vi "shift_register.vi"() -> ()   [LabVIEW 2020]
panel:
  out "Cluster":cluster{"array bool":bool[], "array num":dbl[]}
  out "Array":bool[](array[boolean])
  out "Boolean 2":bool
  out "concatenated string":string
  out "Numeric 2":u16
  in  "stop":bool
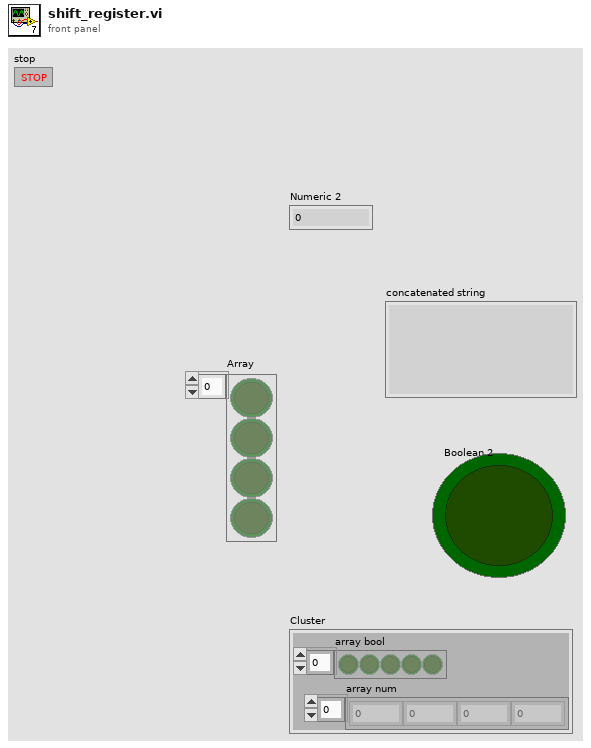
[diagram p1: front panel]
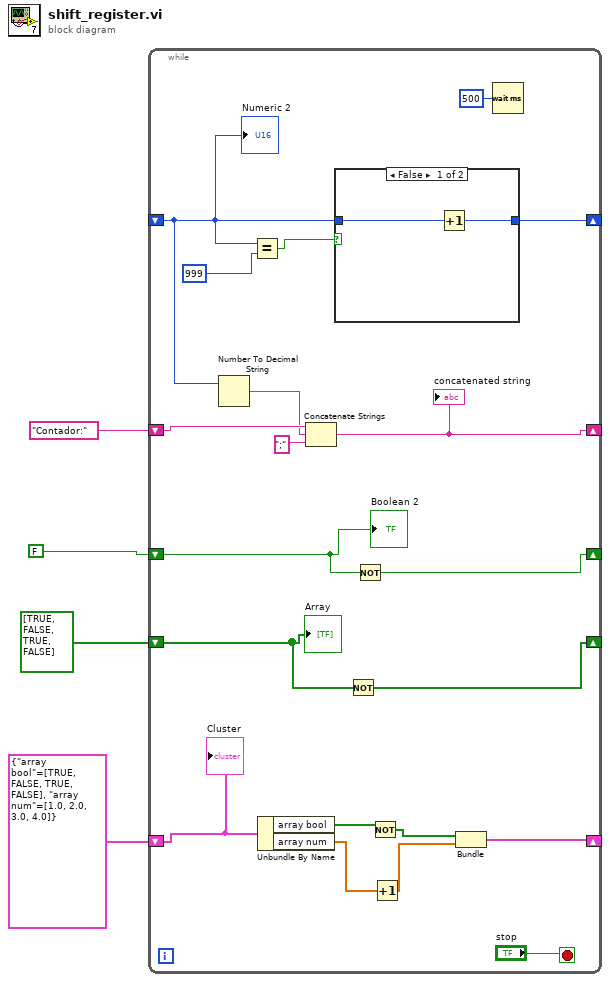
[diagram p0: block diagram]
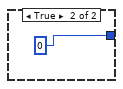
[diagram p2: hidden frame]
diagram:
  n1 = while {
    shift-right: [w22] -> _
    shift-left: _ -> [w19]
    shift-right: [w15] -> _
    shift-left: "Contador:" -> [w18]
    shift-right: [w13] -> _
    shift-left: FALSE -> [w14]
    shift-right: [w12] -> _
    shift-left: bool[] [TRUE, FALSE, TRUE, FALSE] -> [w11]
    shift-right: [w5] -> _
    shift-left: cluster{"array bool":bool[], "array num":dbl[]} {"array bool"=[TRUE, FALSE, TRUE, FALSE], "array num"=[1.0, 2.0, 3.0, 4.0]} -> [w10]
    stop <- "stop" stop-if-true
    n2 = Number To Decimal String(number=w19) -> (decimal integer string=w17:string)  [unwired: 1 in]
    n3 = Equal?(x=w19, y=999) -> (x = y?=w21:bool)
    n4 = Unbundle By Name(w10) -> ("array bool"=w9:bool[], "array num"=w8:dbl[])
    n5 = Concatenate Strings(w18, w17, ";") -> (w15:string)
    "concatenated string" <- w15
    n6 = case shown="False" w21 {
      tunnel: w19 -> [w26 _]
      tunnel: [w25 0] -> w22
      frame False {
        n7 = Increment(x=w26) -> (x+1=w25:i32)
      }
      frame True {
      }
    }
    n8 = Not(x=w11) -> (.not. x?=w12:bool[])
    n9 = Not(x=w14) -> (.not. x?=w13:bool)
    n10 = Not(x=w9) -> (.not. x?=w7:bool[])
    n11 = Increment(x=w8) -> (x+1=w6:dbl[])
    n12 = Bundle(w7, w6) -> (w5:cluster{bool[], dbl[]})  [unwired: 1 in]
    n13 = Wait (ms)(milliseconds to wait=u32 500) -> ()  [unwired: 1 out]
    "Numeric 2" <- w19
    "Boolean 2" <- w14
    "Array" <- w11
    "Cluster" <- w10
  }
